vi "write HRs.vi"(8 "error in (no error)":errorcluster, 10 "values":u16[](array[numeric]), 11 "starting address":u16) -> (0 "error out":errorcluster)   [LabVIEW 2016, in "环境动力监测库.lvlib" / "浮标电源管理.lvlib"]
uses:
  <vilib>/Plasmionique/MB Master/MB Master.lvlib
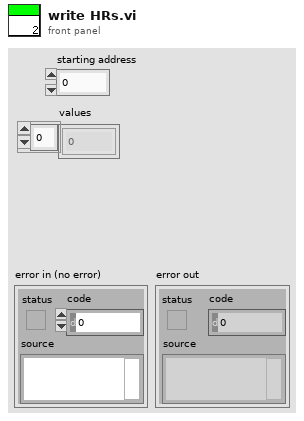
[diagram p1: front panel]
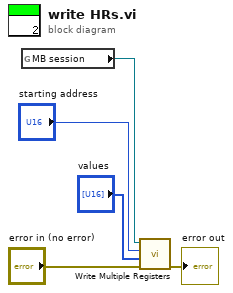
[diagram p0: block diagram]
diagram:
  n1 = global read "通讯全局变量.vi" "MB session"() -> (w5:refnum<class "MB_Master.lvclass">)
  n2 = call <vilib>:"Write Multiple Registers.vi"("error in (no error)"="error in (no error)", "values"="values", "starting address"="starting address", "MB session in"=w5) -> ("error out"=→"error out":errorcluster)  [unwired: 6 in, 1 out]
